vi "get piece from cube  2.vi"() -> ()   [LabVIEW 2018]
uses:
  vision/vision info 2.vi
panel:
  in  "y_plus":dbl
  in  "x_plus":dbl
  in  "grip":bool
  in  "base":i32(slide) scale=-125.0..125.0
  in  "c1":i8
  in  "c2":i8
  in  "camera mode":bool
  in  "z1":dbl
  in  "z2":dbl
  in  "step":dbl
  in  "speed 1":i32
  in  "take":bool
  in  "move":bool
  out "_x":dbl
  out "_y":dbl
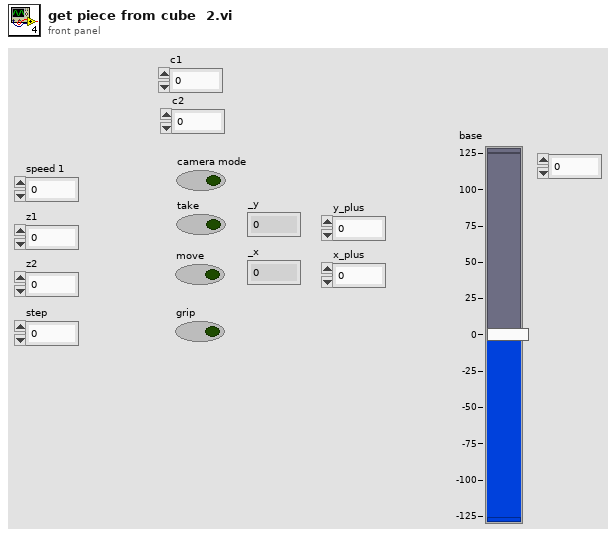
[diagram p1: front panel]
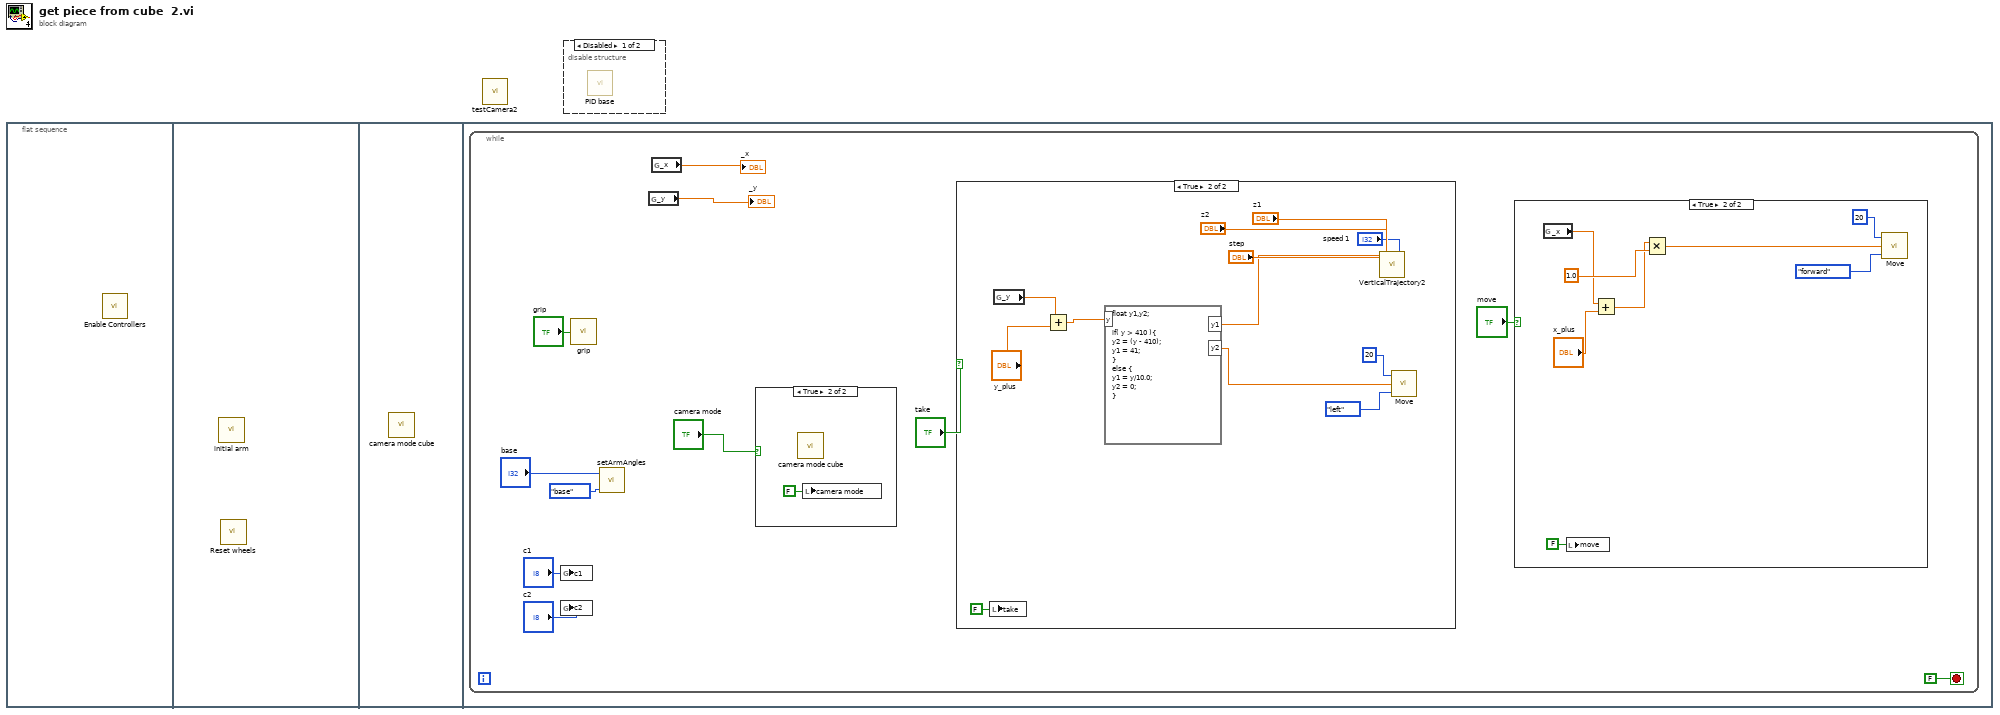
[diagram p0: block diagram]
diagram:
  n1 = flat-sequence {
    frame #0 {
      n2 = call "Enable Controllers.vi"() -> ()  [unwired: 12 in]
    }
    frame #1 {
      n3 = call "initial arm.vi"() -> ()  [unwired: 12 in]
      n4 = call "Reset wheels.vi"() -> ()  [unwired: 12 in]
    }
    frame #2 {
      n5 = call "camera mode cube.vi"() -> ()  [unwired: 12 in]
    }
    frame #3 {
      n6 = while {
        stop <- FALSE stop-if-true
        n7 = global write "vision info 2.vi" "c1"("c1") -> ()
        n8 = global write "vision info 2.vi" "c2"("c2") -> ()
        n9 = call "grip.vi"("grip"="grip") -> ()
        n10 = call "setArmAngles.vi"("Enum"=enum16{"shoulder", "elbow", "wrist", "base"}."base", "angle"="base") -> ()  [unwired: 2 in]
        n11 = global read "vision info 2.vi" "_y"() -> (→"_y":dbl)
        n12 = global read "vision info 2.vi" "_x"() -> (→"_x":dbl)
        n13 = case shown="True" "camera mode" {
          frame False {
          }
          frame True {
            n14 = call "camera mode cube.vi"() -> ()  [unwired: 12 in]
            n15 = local write "camera mode"(FALSE ("camera mode")) -> ()
          }
        }
        n16 = case shown="True" "take" {
          frame False {
          }
          frame True {
            n17 = local write "take"(FALSE ("take")) -> ()
            n18 = global read "vision info 2.vi" "_y"() -> (w26:dbl)
            n19 = Add(x=w26, y="y_plus") -> (x+y=w20:dbl)
            n20 = formula code="float y1,y2;\n\nif( y > 410 ){\ny2 = (y - 410);\ny1 = 41;\n}\nelse {\ny1 = y/10.0;\ny2 = 0;\n}"("y"=w20) -> ("y1"=w22:dbl, "y2"=w21:dbl)
            n21 = call "VerticalTrajectory2.vi"("speed 1"="speed 1", "step"="step", "z2"="z2", "z1"="z1", "x"=w22) -> ()  [unwired: 3 in]
            n22 = call "Move.vi"("Enum"=enum16{"forward", "backward", "left", "right"}."left", "distance"=w21, "speed"=20) -> ()  [unwired: 1 in]
          }
        }
        n23 = case shown="True" "move" {
          frame False {
          }
          frame True {
            n24 = global read "vision info 2.vi" "_x"() -> (w14:dbl)
            n25 = local write "move"(FALSE ("move")) -> ()
            n26 = Add(x=w14, y="x_plus") -> (x+y=w13:dbl)
            n27 = Multiply(x=w13, y=1.0) -> (x*y=w15:dbl)
            n28 = call "Move.vi"("Enum"=enum16{"forward", "backward", "left", "right"}."forward", "distance"=w15, "speed"=20) -> ()  [unwired: 1 in]
          }
        }
      }
    }
  }
  n29 = call "testCamera2.vi"() -> ()  [unwired: 12 in]
  n30 = disable-structure shown="Disabled" {
    frame Disabled {
      n31 = call "PID base.vi"() -> ()  [unwired: 12 in]
    }
    frame Enabled {
    }
  }
